vi "FP midbrain ACT.vi"(0 "Forebrain ACT":dbl[](array[numeric]), 1 "Behavior arrays":T1, 2 "Behavior\nVelocity":dbl=20.0, 3 "error in":errorcluster, 4 "Don't use Forebrain ACT?":bool) -> (5 "Waveform Graph":cluster{dbl, dbl, dbl[]}(graph), 6 "Act Com":T2, 7 "error out":errorcluster)   [LabVIEW 2014]
doc: "This vi is the midbrain ACT routine."
panel:
  out "Max value":dbl
  out "Peak Heading":dbl
  out "Desired\nSpeed":dbl format="%#_13g"
  out "Desired \nRudder":dbl format="%#_13g"
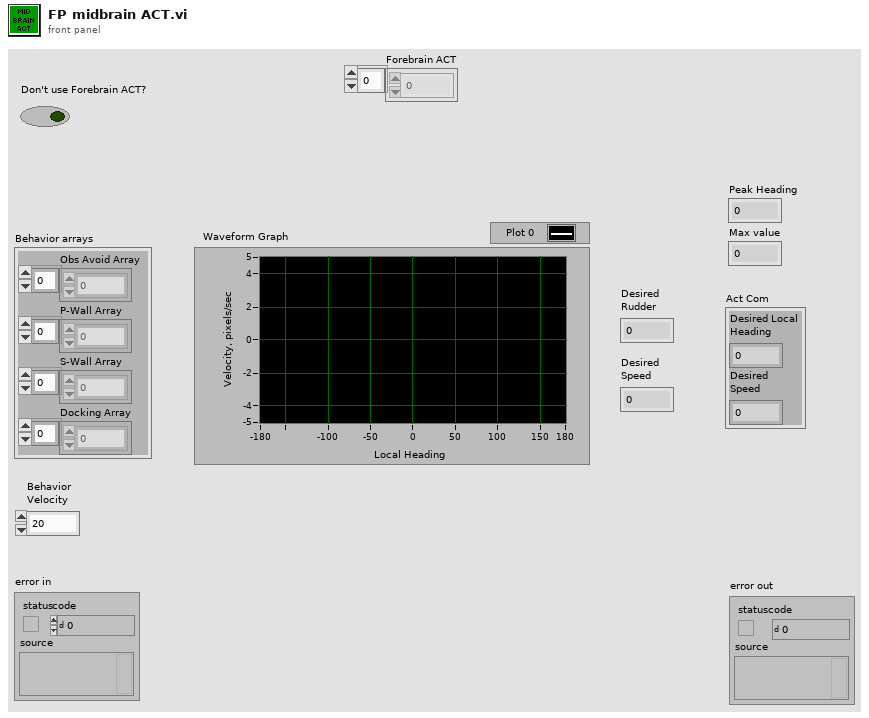
[diagram p1: front panel]
types:
  T1 = cluster{"Obs Avoid Array":dbl[], "P-Wall Array":dbl[], "S-Wall Array":dbl[], "Docking Array":dbl[]}
  T2 = cluster{"Desired Local\nHeading":dbl, "Desired\nSpeed":dbl}
  T3 = cluster{"Peak Heading":dbl, "Behavior\nVelocity":dbl}
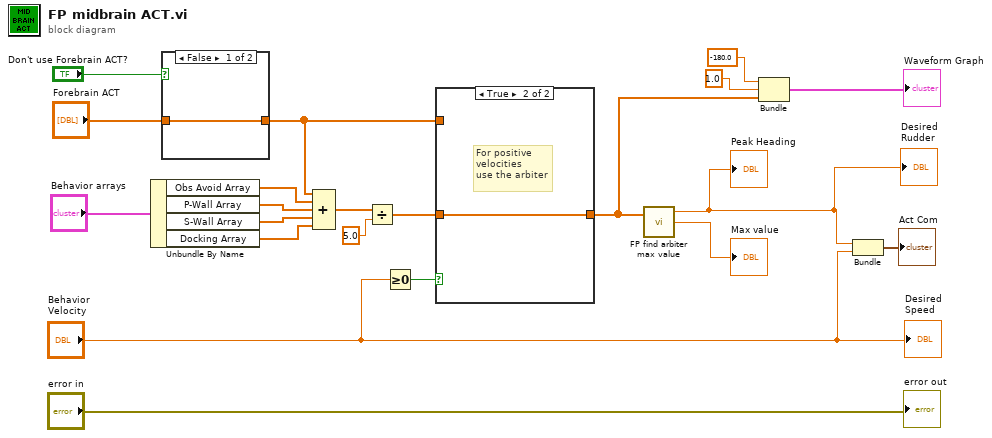
[diagram p0: block diagram]
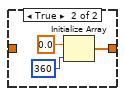
[diagram p2: hidden frame]
diagram:
  n1 = Unbundle By Name("Behavior arrays") -> ("Obs Avoid Array"=w19:dbl[], "P-Wall Array"=w18:dbl[], "S-Wall Array"=w17:dbl[], "Docking Array"=w16:dbl[])
  n2 = case shown="False" "Don't use Forebrain ACT?" {
    tunnel: "Forebrain ACT" -> [w22 _]
    tunnel: [w22 w23] -> w1
    frame False {
    }
    frame True {
      n3 = Initialize Array(0.0 ("element"), 360 ("dimension size")) -> (w23:dbl[])
    }
  }
  n4 = Compound Arithmetic op=ADD(w1, w19, w18, w17, w16) -> (w15:dbl[])
  n5 = Divide(x=w15, y=5.0) -> (x/y=w5:dbl[])
  n6 = Greater Or Equal To 0?(x="Behavior\nVelocity") -> (x >= 0?=w7:bool)
  n7 = case shown="True" w7 {
    tunnel: w5 -> [_ w27]
    tunnel: [w26 w27] -> w4
    tunnel: w1 -> [w26 _]
    frame False {
      # "If velocity is negative\ndo use the arbiter\njust the Forebrain"
    }
    frame True {
      # "For positive \nvelocities\nuse the arbiter"
    }
  }
  n8 = call "FP find arbiter max value.vi"("ACT array"=w4) -> ("Peak Heading"=w8:dbl, "Max value"=→"Max value":dbl)  [unwired: 1 in, 1 out]
  "Desired \nRudder" <- w8
  "Peak Heading" <- w8
  n9 = Bundle(-180.0, 1.0, "Forebrain ACT"=w4) -> (→"Waveform Graph":cluster{dbl, dbl, "Forebrain ACT":dbl[]})  [unwired: 1 in]
  n10 = Bundle("Peak Heading"=w8, "Behavior\nVelocity"="Behavior\nVelocity") -> (→"Act Com":T3)  [unwired: 1 in]
  "Desired\nSpeed" <- "Behavior\nVelocity"
  "error out" <- "error in"
